vi "Do Request.vi"(7 "Processing In":refnum<class "Processing.lvclass">, 11 "PublishConfigController in":refnum<class "PublishConfigController.lvclass">) -> (0 "error out":errorcluster, 5 "Processing":refnum<class "Processing.lvclass">)   [LabVIEW 2020, in "Vecto.lvlib" / "PublishConfigController.lvclass"]
uses:
  PublishConfigController.lvclass
  lv-http-server/HTTP Server/Processing/Processing.lvclass
  RemoteDataService/RemoteDataService.lvclass
  ChannelService/ChannelService.lvclass
  Group/Group.lvclass
  Group Config/Group Config.lvclass
  Channel Config/Channel Config.lvclass
  Publish Config.ctl
  Vecto.lvlib
  Publish Config Response Group.ctl
  Publish Config Response.ctl
  lv-http-util/HTTP Utils/Response/Response.lvclass
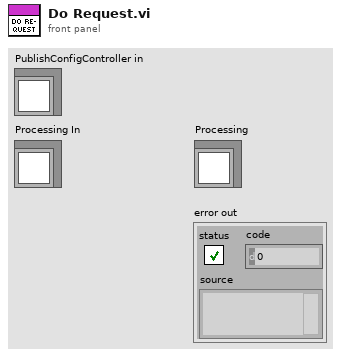
[diagram p1: front panel]
types:
  T1 = typedef "Vecto.lvlib/Publish Config Response.ctl" = cluster{"Groups":T2[]}
  T2 = typedef "Vecto.lvlib/Publish Config Response Group.ctl" = cluster{"Name":string, "Endpoint":T3, "Channels":string[], "OwningTask":string}
  T3 = typedef "Vecto.lvlib/Publish Config.ctl" = cluster{"Address":string, "Port":u16}
  T4 = typedef "Vecto.lvlib/Channel Info.ctl" = cluster{"Name":string, "Group":string, "Owning Node":string, "Owning Task":string, "Resource":string}
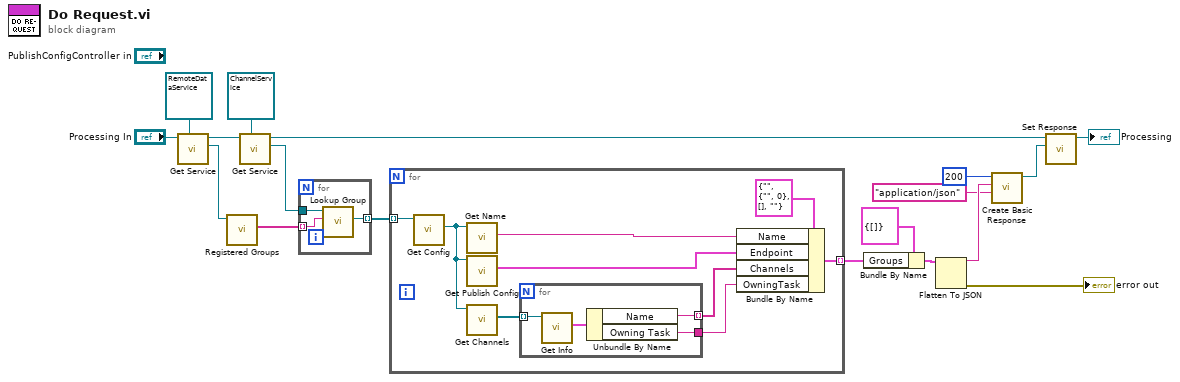
[diagram p0: block diagram]
diagram:
  n1 = call "Get Service.vi"("Service Type"=refnum<class "RemoteDataService.lvclass"> refnum ("Vecto.lvlib:RemoteDataService.lvclass"), "Processing in"="Processing In") -> ("Service"=w16:refnum<class "RemoteDataService.lvclass">, "Processing out"=w15:refnum<class "Processing.lvclass">)  [unwired: 7 in, 1 out]
  n2 = call "Registered Groups.vi"("RemoteDataService in"=w16) -> ("Registered Groups"=w13:string[])  [unwired: 8 in, 2 out]
  n3 = call "Get Service.vi"("Service Type"=refnum<class "ChannelService.lvclass"> refnum ("Vecto.lvlib:ChannelService.lvclass"), "Processing in"=w15) -> ("Service"=w12:refnum<class "ChannelService.lvclass">, "Processing out"=w2:refnum<class "Processing.lvclass">)  [unwired: 7 in, 1 out]
  n4 = for {
    tunnel: w13 -> [w21] mode=indexing
    tunnel: w12 -> [w20]
    tunnel: [w19] -> w11 mode=indexing
    n5 = call "Lookup Group.vi"("Group Name"=w21, "ChannelService in"=w20) -> ("Group"=w19:refnum<class "Group.lvclass">)  [unwired: 7 in, 2 out]
  }
  n6 = for {
    tunnel: w11 -> [w30] mode=indexing
    tunnel: [w22] -> w9 mode=indexing
    n7 = call "Get Config.vi"("Group in"=w30) -> ("Config"=w29:refnum<class "Group Config.lvclass">)  [unwired: 8 in, 2 out]
    n8 = call "Get Name.vi"("Group Config in"=w29) -> ("Name"=w26:string)  [unwired: 8 in, 2 out]
    n9 = call "Get Publish Config.vi"("Group Config in"=w29) -> ("Publish Config"=w25:T3)  [unwired: 8 in, 2 out]
    n10 = call "Get Channels.vi"("Group Config in"=w29) -> ("Channels"=w28:refnum<class "Channel Config.lvclass">[])  [unwired: 8 in, 2 out]
    n11 = for {
      tunnel: w28 -> [w34] mode=indexing
      tunnel: [w32] -> w24 mode=indexing
      tunnel: [w31] -> w23
      n12 = call "Get Info.vi"("Channel Config in"=w34) -> ("Info"=w33:T4)  [unwired: 8 in, 2 out]
      n13 = Unbundle By Name(w33) -> ("Name"=w32:string, "Owning Task"=w31:string)
    }
    n14 = Bundle By Name(cluster=T2 {"Name"="", "Endpoint"={"Address"="", "Port"=0}, "Channels"=[], "OwningTask"=""} ("Publish Config Group"), "Name"=w26, "Endpoint"=w25, "Channels"=w24, "OwningTask"=w23) -> (w22:T2)
  }
  n15 = Bundle By Name(cluster=T1 {"Groups"=[]} ("Publish Config Response"), "Groups"=w9) -> (w8:T1)
  n16 = Flatten To JSON(anything=w8) -> (JSON string=w6:string, 11:→"error out":errorcluster)  [unwired: 2 in]
  n17 = call "Create Basic Response.vi"("Content-Type (text/plain)"="application/json", "Payload"=w6, "Status Code"=u16 200) -> ("Response out"=w3:refnum<class "Response.lvclass">)  [unwired: 7 in, 1 out]
  n18 = call "Set Response.vi"("Response"=w3, "Processing in"=w2) -> ("Processing out"=→"Processing":refnum<class "Processing.lvclass">)  [unwired: 9 in]
